vi "Format_graph_fields.vi"(2 "error out 2":errorcluster, 3 "appended array 2":refnum<vi>[](array[refnum]), 4 "report out 2":refnum<class "NI_report.lvclass">) -> (0 "error out":errorcluster, 1 "report out":refnum<class "NI_report.lvclass">)   [LabVIEW 2010]
uses:
  <vilib>/Utility/NIReport.llb/NI_report.lvclass
  <vilib>/Utility/miscctls.llb/LVBoundsTypeDef.ctl
  <vilib>/Utility/NIReport.llb/HTML Report Image Alignment.ctl
  <vilib>/Utility/NIReport.llb/image depth.ctl
  <vilib>/picture/picture.llb/Draw True-Color Pixmap.vi
  <vilib>/Utility/NIReport.llb/Append Report Text (str wrap).vi
  <vilib>/Utility/NIReport.llb/NI_ReportGenerationCore.lvlib
panel:
  out "Draw Area Size":T1
  out "2D Picture":picture
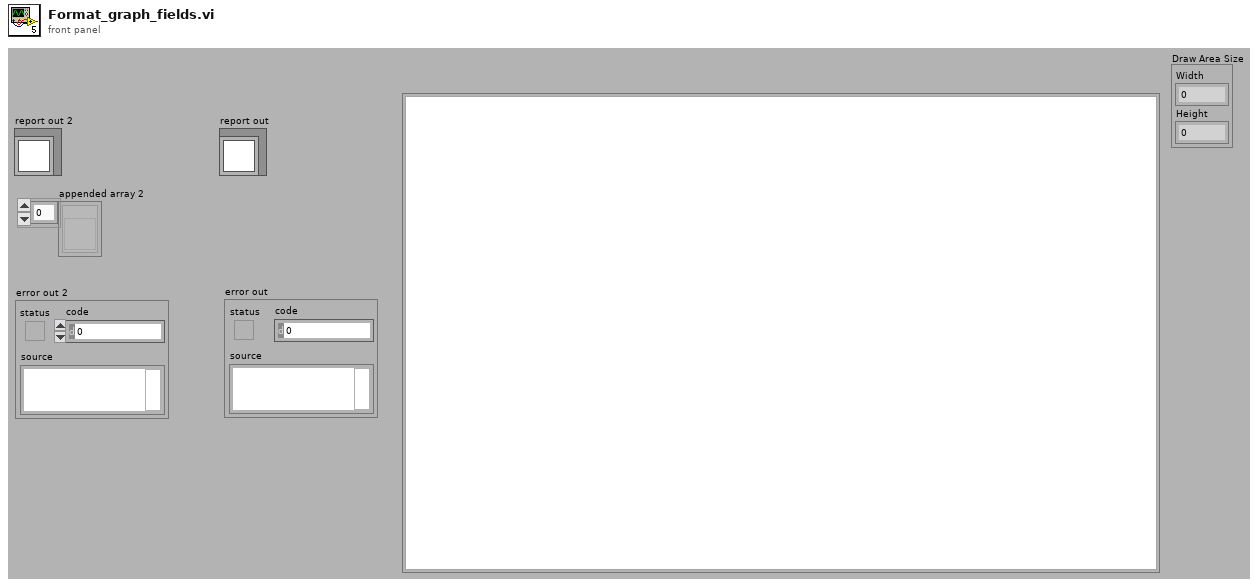
[diagram p1: front panel]
types:
  T1 = typedef "LVBoundsTypeDef.ctl" = cluster{"Width":u32, "Height":u32}
  T2 = cluster{"position (Excel)":cluster{"row":i32, "column":i32}, "name (Excel)":string, "bookmark (Word)":string}
  T3 = typedef "imagedata.ctl" = cluster{"image type":i32, "image depth":i32, "image":u8[], "mask":u8[], "colors":u32[], "Rectangle":cluster{"left":i16, "top":i16, "right":i16, "bottom":i16}}
  T4 = typedef "NI_ReportGenerationCore.lvlib/HTML Report Image Alignment.ctl" = enum16{"(default)", "LEFT", "RIGHT", "TOP", "TEXTTOP", "MIDDLE", "ABSMIDDLE", "BASELINE", "BOTTOM", "ABSBOTTOM"}
  T5 = typedef "NI_ReportGenerationCore.lvlib/image depth.ctl" = u16
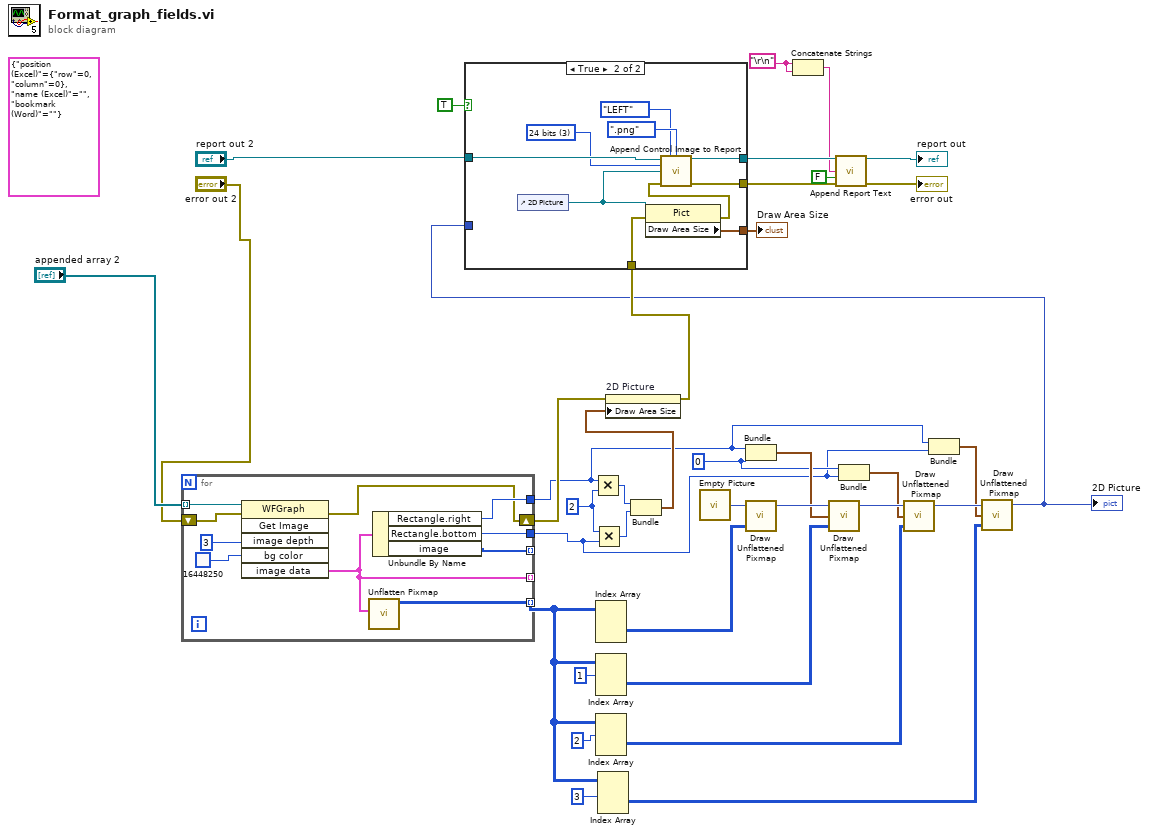
[diagram p0: block diagram]
diagram:
  w3 = "\r\n"
  (unwired) T2 {"position (Excel)"={"row"=0, "column"=0}, "name (Excel)"="", "bookmark (Word)"=""} ("MS Office parameters")
  w18 = 0
  w36 = 2
  n1 = for {
    tunnel: "appended array 2" -> [w46] mode=indexing
    tunnel: [w39] -> _ mode=indexing
    tunnel: [w45] -> w16
    tunnel: [w44] -> w15
    tunnel: [w43] -> _ mode=indexing
    tunnel: [w38] -> w13 mode=indexing
    shift-right: [w41] -> w26
    shift-left: "error out 2" -> [w42]
    n2 = invoke class="WFGraph" method="Get Image"(reference=w46, error in=w42, "image depth"=3 ("Image Depth"), "bg color"=u32 16448250) -> (error out=w41:errorcluster, "image data"=w39:T3)  [unwired: 2 in, 4 out]
    n3 = call <vilib>:"Unflatten Pixmap.vi"("image data"=w39) -> ("24-bit pixmap"=w38:u32[][])  [unwired: 4 in, 6 out]
    n4 = Unbundle By Name(w39) -> ("Rectangle.right"=w45:i16, "Rectangle.bottom"=w44:i16, "image"=w43:u8[])
  }
  n5 = Multiply(x=w16, y=w36) -> (x*y=w28:i32)
  n6 = Multiply(x=w36, y=w15) -> (x*y=w29:i32)
  n7 = Index Array(array=w13) -> (element=w34:u32[][])  [unwired: 3 in]
  n8 = Index Array(array=w13, index (dim 0)=1 ("index (page)")) -> (element=w30:u32[][])  [unwired: 2 in]
  n9 = Index Array(array=w13, index (dim 0)=2 ("index (page)")) -> (element=w22:u32[][])  [unwired: 2 in]
  n10 = Index Array(array=w13, index (dim 0)=3 ("index (page)")) -> (element=w19:u32[][])  [unwired: 2 in]
  n11 = Bundle(w28, w29) -> (w27:cluster{i32, i32})  [unwired: 1 in]
  n12 = property on="2D Picture" class="Pict"(error in=w26, "Draw Area Size"=w27) -> (error out=w25:errorcluster)  [unwired: 1 in, 1 out]
  n13 = call "Empty Picture"() -> ("empty picture"=w35:picture)
  n14 = Bundle("right"=w16, w18) -> (w32:cluster{"right":i16, i32})  [unwired: 1 in]
  n15 = call-poly <vilib>:"Draw Unflattened Pixmap.vi"("picture"=w35, "data (RGB format)"=w34) -> ("new picture"=w33:picture)  [unwired: 7 in]
  n16 = Concatenate Strings(w3, w3) -> (w2:string)
  n17 = call-poly <vilib>:"Draw Unflattened Pixmap.vi"("picture"=w33, "top left point(0, 0)"=w32, "data (RGB format)"=w30) -> ("new picture"=w21:picture)  [unwired: 6 in]
  n18 = Bundle(w18, "bottom"=w15) -> (w17:cluster{i32, "bottom":i16})  [unwired: 1 in]
  n19 = call-poly <vilib>:"Draw Unflattened Pixmap.vi"("picture"=w21, "top left point(0, 0)"=w17, "data (RGB format)"=w22) -> ("new picture"=w20:picture)  [unwired: 6 in]
  n20 = Bundle("right"=w16, "bottom"=w15) -> (w14:cluster{"right":i16, "bottom":i16})  [unwired: 1 in]
  n21 = call-poly <vilib>:"Draw Unflattened Pixmap.vi"("picture"=w20, "top left point(0, 0)"=w14, "data (RGB format)"=w19) -> ("new picture"=w9:picture)  [unwired: 6 in]
  "2D Picture" <- w9
  n22 = case shown="True" TRUE {
    tunnel: [w48 w59] -> w8
    tunnel: [w49 w58] -> w7
    tunnel: w25 -> [w48 w51]
    tunnel: "report out 2" -> [w49 w57]
    tunnel: w9 -> [_ _]
    tunnel: [_ w52] -> w1
    frame False {
    }
    frame True {
      w55 = T5 3 items=["B&W", "4 bits", "8 bits", "24 bits"] ("image depth")
      n23 = control-ref of="2D Picture"() -> (w53:refnum<vi>)
      n24 = property class="Pict"(reference=w53, error in=w51) -> (error out=w50:errorcluster, "Draw Area Size"=w52:T1)  [unwired: 1 out]
      n25 = call-dynamic "Append Control Image to Report.vi"("report in"=w57, "alignment (default)"=HTML_Report_Image_Alignment."LEFT", "image file type (.jpg)"=enum16{".jpg", ".png"}.".png", "image depth"=w55, "ctrl reference"=w53, "error in (no error)"=w50) -> ("report out"=w58:refnum<class "NI_report.lvclass">, "error out"=w59:errorcluster)  [unwired: 6 in, 2 out]
    }
  }
  "Draw Area Size" <- w1
  n26 = call-poly <vilib>:"Append Report Text.vi"("report in"=w7, "text"=w2, "append on new line? (F)"=FALSE, "error in (no error)"=w8) -> ("report out"=→"report out":refnum<class "NI_report.lvclass">, "error out"=→"error out":errorcluster)  [unwired: 2 in, 8 out]
